vi "Update local DB (SubVI).vi"(4 "error in":errorcluster, 7 "clusterListboxes":T1) -> (0 "error out":errorcluster)   [LabVIEW 2010]
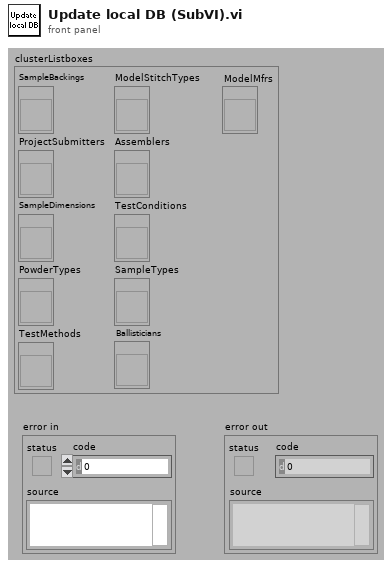
[diagram p1: front panel]
types:
  T1 = cluster{"SampleBackings":refnum<vi>, "ProjectSubmitters":refnum<vi>, "SampleDimensions":refnum<vi>, "PowderTypes":refnum<vi>, "TestMethods":refnum<vi>, "ModelStitchTypes":refnum<vi>, "Assemblers":refnum<vi>, "TestConditions":refnum<vi>, "SampleTypes":refnum<vi>, "Ballisticians":refnum<vi>, "ModelMfrs":refnum<vi>}
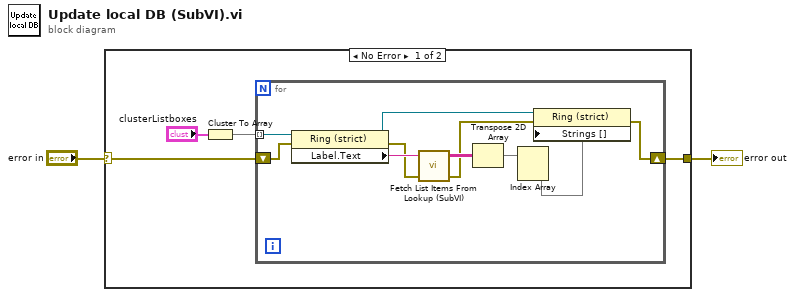
[diagram p0: block diagram]
diagram:
  n1 = case shown="No Error" "error in" {
    selector: "error in" -> [w4 w17]
    tunnel: [w3 w17] -> w1
    frame No Error {
      n2 = Cluster To Array(cluster="clusterListboxes") -> (array=w5:refnum<vi>[])
      n3 = for {
        tunnel: w5 -> [w16] mode=indexing
        shift-right: [w14] -> w3
        shift-left: w4 -> [w15]
        n4 = property class="Ring (strict)"(reference=w16, error in=w15) -> (reference out=w11:refnum<vi>, error out=w12:errorcluster, "Label.Text"=w13:string)
        n5 = call "Fetch List Items From Lookup (SubVI).vi"("error IN"=w12, "Query"=w13) -> ("error OUT"=w9:errorcluster, "recordset data"=w10:string[][])  [unwired: 2 out]
        n6 = Transpose 2D Array(2D array=w10) -> (transposed array=w8:string[][])
        n7 = Index Array(array=w8) -> (element=w7:string[])  [unwired: 2 in]
        n8 = property class="Ring (strict)"(reference=w11, error in=w9, "Strings []"=w7) -> (error out=w14:errorcluster)  [unwired: 1 out]
      }
    }
    frame Error {
    }
  }
  "error out" <- w1
